vi "Grow Datum Array.vi"(2 "size":i32, 3 "bytestream":refnum<class "Bytestream.lvclass">) -> (1 "bytestream out":refnum<class "Bytestream.lvclass">)   [LabVIEW 2020, in "NI_Bytestream.lvlib" / "Bytestream.lvclass"]
uses:
  <vilib>/Array/Bytestream/Bytestream.lvclass
  <vilib>/Array/Bytestream/Bytestream.lvclass/Bytestream.ctl
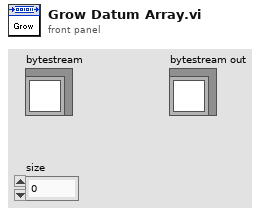
[diagram p1: front panel]
types:
  T1 = typedef "NI_Bytestream.lvlib/Bytestream.lvclass/Datum.ctl" = cluster{"array":u8[], "index":i32}
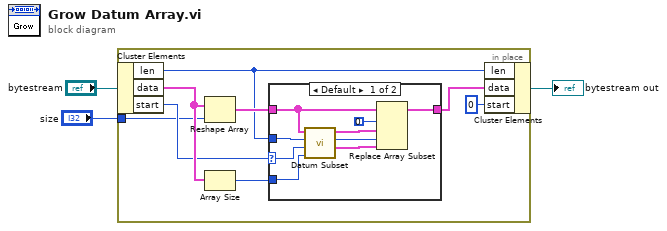
[diagram p0: block diagram]
diagram:
  n1 = in-place {
    in-place-border: "size" -> [w4]
    n2 = in-place-cluster #1("bytestream") -> ("len"=w6:i32, "data"=w10:T1[], "start"=w7:i32)
    n3 = Reshape Array(w10, w4) -> (w9:T1[])
    n4 = Array Size(array=w10) -> (size(s)=w5:i32)
    n5 = case shown="Default" w7 {
      selector: w7 -> [w18 _]
      tunnel: w9 -> [w12 w21]
      tunnel: [w20 w21] -> w8
      tunnel: w6 -> [w19 _]
      tunnel: w5 -> [w13 _]
      frame Default {
        n6 = call <vilib>:"Datum Subset.vi"("limit size"=w13, "start"=w18, "len"=w19, "data"=w12) -> ("datums out"=w14:T1[], "count of datums 1"=w16:i32, "datums 1"=w15:T1[])  [unwired: 4 in, 1 out]
        n7 = Replace Array Subset(array=w12, new element #1=w15, index #1=0 ("index"), new element #2=w14, index #2=w16) -> (w20:T1[])
      }
      frame 0 {
      }
    }
    n8 = in-place-cluster #1("len"=w6, "data"=w8, "start"=0) -> (→"bytestream out":refnum<class "Bytestream.lvclass">)
  }
